vi "Single Class_Multiple_State_Self.vi"(0 "State#":i32=1000, 1 "State_Interval_Time(s)":dbl=0.001 min=0.0 max=86400.0 format="%#_13p", 2 "Time Target (s)":dbl=30.0 format="%#_13g", 3 "System_Delay(s)":dbl=0.01 min=0.0 max=86400.0 format="%#_13p") -> ()   [LabVIEW 2021]
uses:
  C:/Program Files (x86)/Hyper State Machine Framework/SSW_Hyper_State_Machine.lvlibp/State_Machine_Class/Main_State_Machine/Hyper_State_Machine.lvclass
  C:/Program Files (x86)/Hyper State Machine Framework/SSW_Hyper_State_Machine.lvlibp/State_Machine_Class/State_Machine_Module.llb/State Machine[].ctl
  C:/Program Files (x86)/Hyper State Machine Framework/SSW_Hyper_State_Machine.lvlibp/State_Machine_Class/State_Machine_Module.llb/Iterval.ctl
  C:/Program Files (x86)/Hyper State Machine Framework/SSW_Hyper_State_Machine.lvlibp/State_Machine_Class/State_Machine_Module.llb/Lock_Unlock.ctl
  C:/Program Files (x86)/Hyper State Machine Framework/SSW_Hyper_State_Machine.lvlibp
panel:
  out "Current_State_Active":bool
  out "Previous_State_Active":bool
  out "Current State":string
  out "Show_Stop_Button":bool=TRUE
  in  "Unlock":bool
  in  "Reset":bool
  in  "Lock Even":bool
  in  "Lock Odd":bool
  in  "lock All":bool
  in  "Stop":bool
  out "Timing":dbl[](array[numeric])
  out "Lock":bool[](array[boolean])
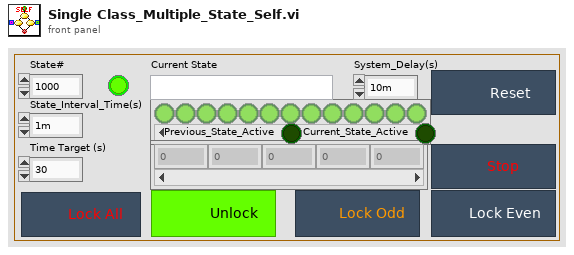
[diagram p1: front panel]
types:
  T1 = typedef "SSW_Hyper_State_Machine.lvlibp/State Machine.ctl" = cluster{"Command":string, "Data":variant}
  T2 = typedef "SSW_Hyper_State_Machine.lvlibp/State Machine[].ctl" = cluster{"Command":string, "Data":variant}[]
  T3 = typedef "SSW_Hyper_State_Machine.lvlibp/Lock_Unlock.ctl" = cluster{"Action_Mode (Get)":enum16{"Set", "Get"}, "Action_Set (False)":bool, "State_In (Wait)":string}
  T4 = typedef "SSW_Hyper_State_Machine.lvlibp/Iterval.ctl" = cluster{"Delay(s)":dbl, "State (Interval_Delay)":string}
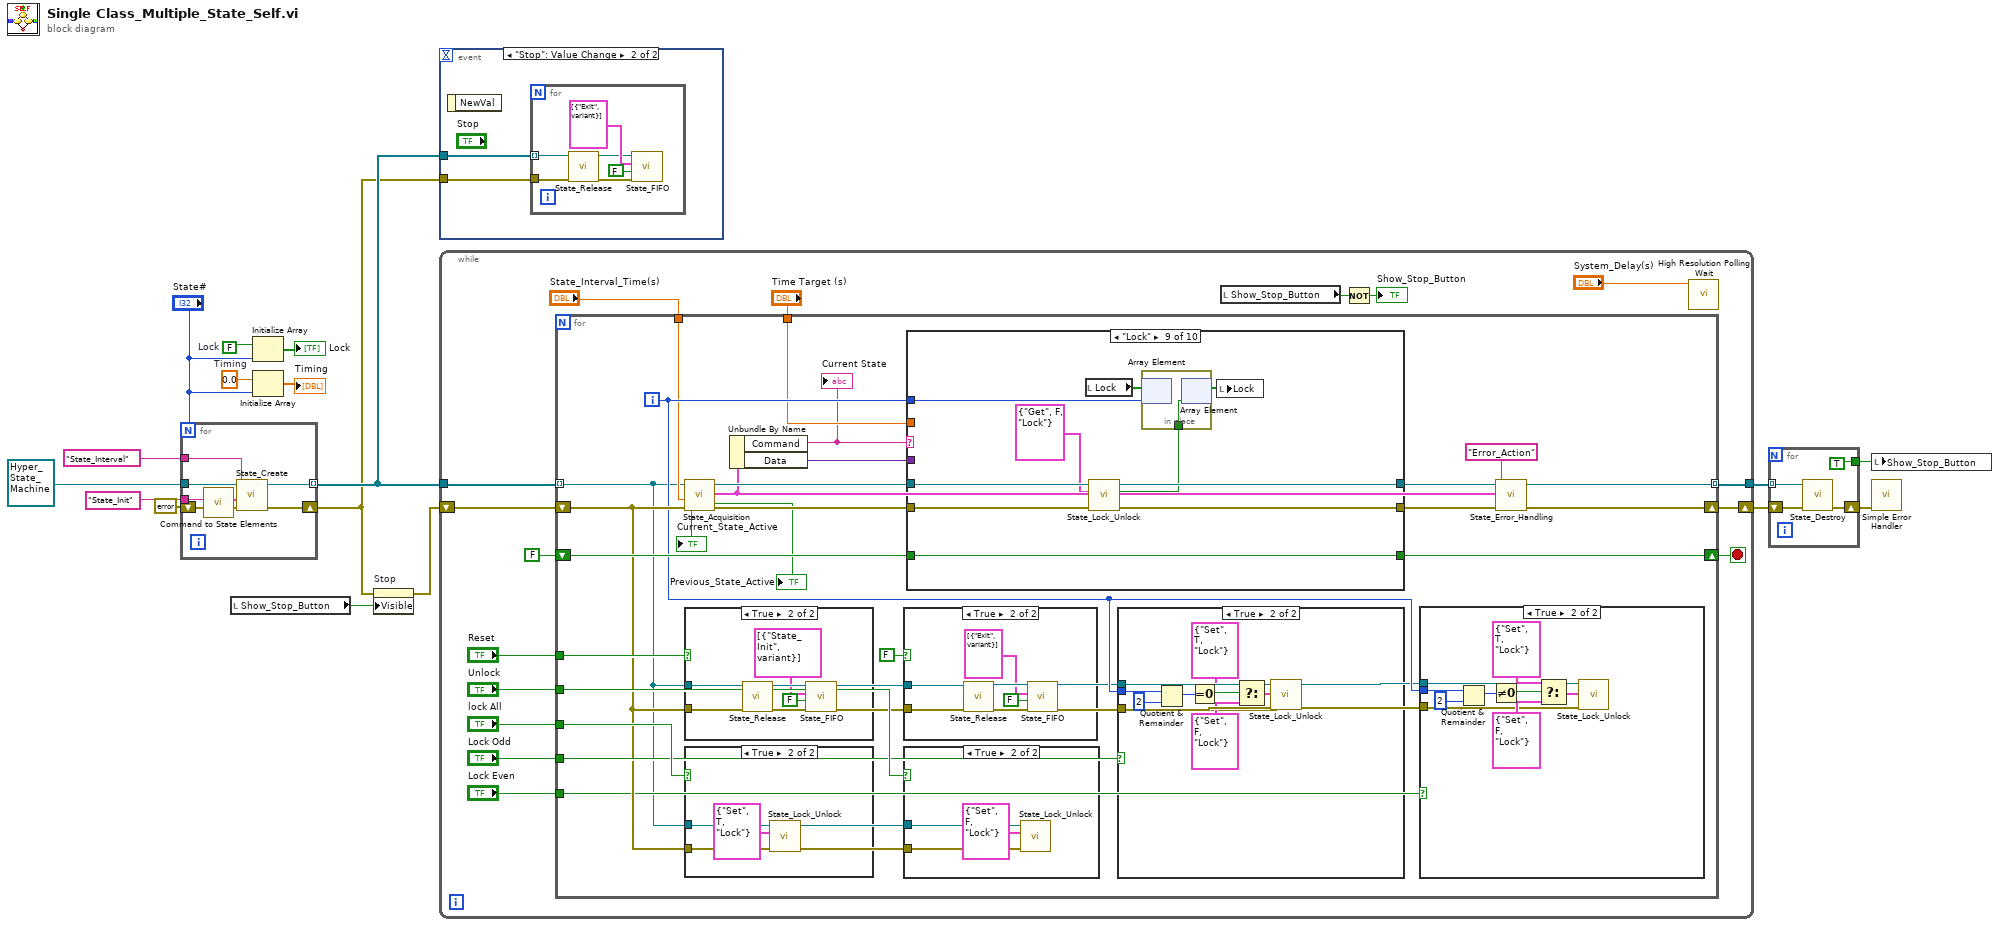
[diagram p0: block diagram]
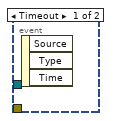
[diagram p2: hidden frame]
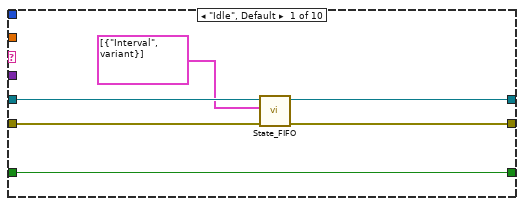
[diagram p9: hidden frame]
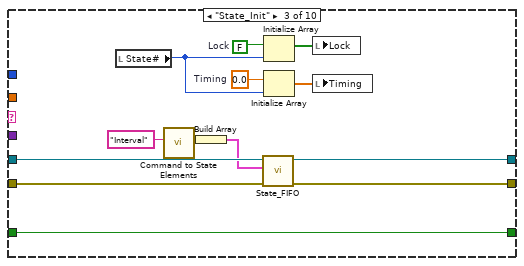
[diagram p11: hidden frame]
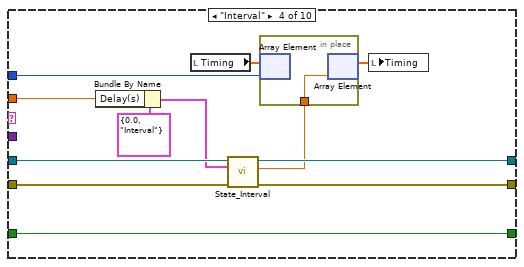
[diagram p12: hidden frame]
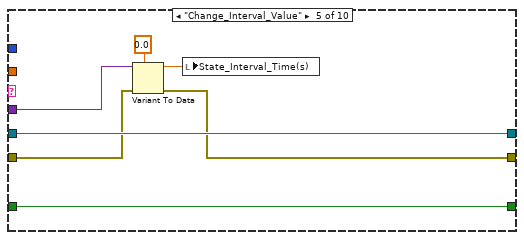
[diagram p13: hidden frame]
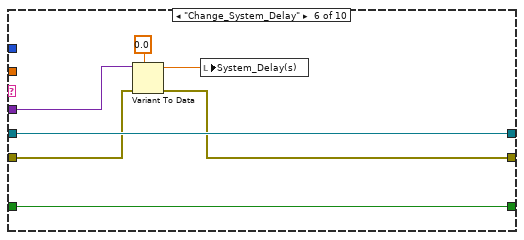
[diagram p14: hidden frame]
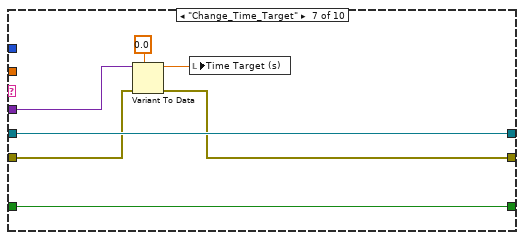
[diagram p15: hidden frame]
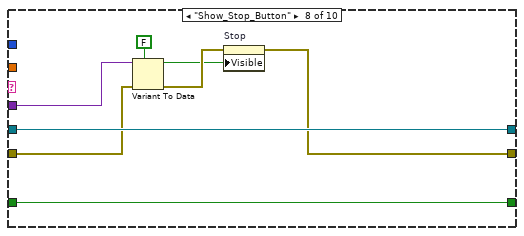
[diagram p16: hidden frame]
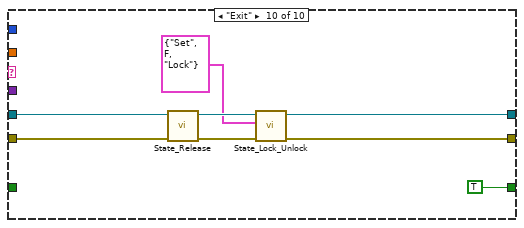
[diagram p17: hidden frame]
diagram:
  w14 = 0.0  # Timing
  w17 = FALSE  # Lock
  n1 = for {
    N: "State#" -> [_]
    tunnel: refnum<class "Hyper_State_Machine.lvclass"> refnum ("SSW_Hyper_State_Machine.lvlibp:Hyper_State_Machine.lvclass") -> [w18]
    tunnel: "State_Init" ("Command") -> [w23]
    tunnel: "State_Interval" ("Core_Interval_Name(State_Interval)") -> [w22]
    shift-right: [w21] -> w5
    shift-left: errorcluster {"status"=FALSE, "code"=0, "source"=""} ("error out") -> [w20]
    tunnel: [w19] -> w6 mode=indexing
    n2 = call "Command to State Elements.vi"("Command"=w23) -> ("Command to State Elements"=w24:T1)  [unwired: 10 in]
    n3 = call-dynamic "State_Create.vi"("error in (no error)"=w20, "Init_State(Option)"=w24, "State_Interval_Name"=w22, "State_Machine_Class in"=w18) -> ("error out"=w21:errorcluster, "State_Machine_Class out"=w19:refnum<class "Hyper_State_Machine.lvclass">)  [unwired: 5 in, 1 out]
  }
  n4 = local read "Show_Stop_Button"() -> (w8:bool)
  n5 = Initialize Array(w17, "State#") -> (→"Lock":bool[])
  n6 = Initialize Array(w14, "State#") -> (→"Timing":dbl[])
  n7 = property on="Stop" class="Bool"(error in=w5, "Visible"=w8) -> (error out=w9:errorcluster)  [unwired: 1 in, 1 out]
  n8 = event shown="[1] \"Stop\": Value Change" {
    selector: _ -> [_ _]
    dyn-events: _ -> [_ _]
    timeout: _ -> [_ _]
    tunnel: w6 -> [_ w26]
    tunnel: w5 -> [_ w25]
    event Timeout {
      n9 = event-data() -> ()  [unwired: 1 in, 3 out]
    }
    event "Stop": Value Change {
      n10 = event-data() -> ()  [unwired: 1 in, 1 out]
      n11 = for {
        tunnel: w26 -> [w28] mode=indexing
        tunnel: w25 -> [w27]
        n12 = call-dynamic "State_Release.vi"("error in (no error)"=w27, "State_Machine_Class in"=w28) -> ("error out"=w30:errorcluster, "State_Machine_Class out"=w29:refnum<class "Hyper_State_Machine.lvclass">)  [unwired: 8 in]
        n13 = call-dynamic "State_FIFO.vi"("error in (no error)"=w30, "State_Interval(Enable)"=FALSE, "State Machine[]"=T2 [{"Command"="Exit", "Data"=variant}], "State_Machine_Class in"=w29) -> ()  [unwired: 6 in, 2 out]
      }
    }
  }
  n14 = while {
    tunnel: w6 -> [w48]
    tunnel: [w44] -> w11
    shift-right: [w43] -> w10
    shift-left: w9 -> [w47]
    stop <- w46 stop-if-true
    n15 = for {
      tunnel: w48 -> [w49] mode=indexing
      shift-right: [w70] -> w43
      shift-left: w47 -> [w58]
      shift-right: [w65] -> w46
      shift-left: FALSE -> [w64]
      tunnel: [w63] -> w44 mode=indexing
      tunnel: "Reset" -> [w62]
      tunnel: "lock All" -> [w61]
      tunnel: "Unlock" -> [w60]
      tunnel: "Lock Odd" -> [w59]
      tunnel: "Lock Even" -> [w57]
      tunnel: "Time Target (s)" -> [w55]
      tunnel: "State_Interval_Time(s)" -> [w54]
      i -> [w56]
      n16 = call-dynamic "State_Acquisition.vi"("error in (no error)"=w58, "State_Interval_Time(s)"=w54, "Main_Machine_State_Class in"=w49) -> ("error out"=w71:errorcluster, "State"=w69:T1, "Main_Machine_State_Class out"=w72:refnum<class "Hyper_State_Machine.lvclass">, "Previous_State_Active"=→"Previous_State_Active":bool, "Current_State_Active"=→"Current_State_Active":bool)  [unwired: 2 in, 2 out]
      n17 = case shown="True" w62 {
        tunnel: w49 -> [_ w109]
        tunnel: w58 -> [_ w105]
        frame False {
        }
        frame True {
          n18 = call-dynamic "State_Release.vi"("error in (no error)"=w105, "State_Machine_Class in"=w109) -> ("error out"=w107:errorcluster, "State_Machine_Class out"=w108:refnum<class "Hyper_State_Machine.lvclass">)  [unwired: 8 in]
          n19 = call-dynamic "State_FIFO.vi"("error in (no error)"=w107, "State_Interval(Enable)"=FALSE, "State Machine[]"=T2 [{"Command"="State_Init", "Data"=variant}], "State_Machine_Class in"=w108) -> ()  [unwired: 6 in, 2 out]
        }
      }
      n20 = case shown="True" w61 {
        tunnel: w49 -> [_ w97]
        tunnel: w58 -> [_ w96]
        frame False {
        }
        frame True {
          n21 = call-dynamic "State_Lock_Unlock.vi"("error in (no error)"=w96, "Parameter"=T3 {"Action_Mode (Get)"=enum."Set", "Action_Set (False)"=TRUE, "State_In (Wait)"="Lock"}, "State_Machine_Class in"=w97) -> ()  [unwired: 6 in, 3 out]
        }
      }
      n22 = Unbundle By Name(w69) -> ("Command"=w52:string, "Data"=w73:variant)
      "Current State" <- w52
      n23 = case shown="True" FALSE {
        tunnel: w49 -> [_ w103]
        tunnel: w58 -> [_ w99]
        frame False {
        }
        frame True {
          n24 = call-dynamic "State_Release.vi"("error in (no error)"=w99, "State_Machine_Class in"=w103) -> ("error out"=w101:errorcluster, "State_Machine_Class out"=w102:refnum<class "Hyper_State_Machine.lvclass">)  [unwired: 8 in]
          n25 = call-dynamic "State_FIFO.vi"("error in (no error)"=w101, "State_Interval(Enable)"=FALSE, "State Machine[]"=T2 [{"Command"="Exit", "Data"=variant}], "State_Machine_Class in"=w102) -> ()  [unwired: 6 in, 2 out]
        }
      }
      n26 = case shown="True" w60 {
        tunnel: w49 -> [_ w93]
        tunnel: w58 -> [_ w94]
        frame False {
        }
        frame True {
          n27 = call-dynamic "State_Lock_Unlock.vi"("error in (no error)"=w94, "Parameter"=T3 {"Action_Mode (Get)"=enum."Set", "Action_Set (False)"=FALSE, "State_In (Wait)"="Lock"}, "State_Machine_Class in"=w93) -> ()  [unwired: 6 in, 3 out]
        }
      }
      n28 = case shown="\"Lock\"" w52 {
        tunnel: w73 -> [_ _ _ _ w150 w157 w164 w172 _ _]
        tunnel: w72 -> [w114 w118 w130 w137 w151 w158 w165 w173 w183 w191]
        tunnel: w71 -> [w113 w117 w128 w136 w149 w156 w163 w171 w182 w190]
        tunnel: [w112 w118 w129 w134 w151 w158 w165 w173 w181 w187] -> w67
        tunnel: [w111 w117 w127 w133 w148 w155 w162 w166 w180 w186] -> w66
        tunnel: w56 -> [_ _ _ w143 _ _ _ _ w176 _]
        tunnel: [w115 w116 w131 w140 w146 w153 w160 w170 w178 TRUE] -> w65
        tunnel: w64 -> [w115 w116 w131 w140 w146 w153 w160 w170 w178 _]
        tunnel: w55 -> [_ _ _ w139 _ _ _ _ _ _]
        frame "Idle", Default {
          n29 = call-dynamic "State_FIFO.vi"("error in (no error)"=w113, "State Machine[]"=T2 [{"Command"="Interval", "Data"=variant}], "State_Machine_Class in"=w114) -> ("error out"=w111:errorcluster, "State_Machine_Class out"=w112:refnum<class "Hyper_State_Machine.lvclass">)  [unwired: 7 in]
        }
        frame "State_Interval" {
          # "Execute Every Define of State Interval Time"
        }
        frame "State_Init" {
          w123 = 0.0  # Timing
          w122 = FALSE  # Lock
          n30 = local read "State#"() -> (w121:i32)
          n31 = call "Command to State Elements.vi"("Command"="Interval") -> ("Command to State Elements"=w125:T1)  [unwired: 10 in]
          n32 = Build Array(w125) -> (w124:T1[])
          n33 = call-dynamic "State_FIFO.vi"("error in (no error)"=w128, "State Machine[]"=w124, "State_Machine_Class in"=w130) -> ("error out"=w127:errorcluster, "State_Machine_Class out"=w129:refnum<class "Hyper_State_Machine.lvclass">)  [unwired: 7 in]
          n34 = Initialize Array(w122, w121) -> (w119:bool[])
          n35 = Initialize Array(w123, w121) -> (w120:dbl[])
          n36 = local write "Lock"(w119) -> ()
          n37 = local write "Timing"(w120) -> ()
        }
        frame "Interval" {
          n38 = Bundle By Name(cluster=T4 {"Delay(s)"=0.0, "State (Interval_Delay)"="Interval"} ("Parameter"), "Delay(s)"=w139) -> (w135:T4)
          n39 = local read "Timing"() -> (w142:dbl[])
          n40 = call-dynamic "State_Interval.vi"("error in (no error)"=w136, "Parameter"=w135, "State_Machine_Class in"=w137) -> ("error out"=w133:errorcluster, "Elapsed Time(s)"=w132:dbl, "State_Machine_Class out"=w134:refnum<class "Hyper_State_Machine.lvclass">)  [unwired: 6 in]
          n41 = in-place {
            in-place-border: w132 -> [w144]
            n42 = in-place-array #1(w142, w143) -> ()  [unwired: 1 out]
            n43 = in-place-array #1(w144) -> (w141:dbl[])  [unwired: 1 out]
          }
          n44 = local write "Timing"(w141) -> ()
        }
        frame "Change_Interval_Value" {
          n45 = Variant To Data(error in=w149, type=0.0 ("Time Target (s)"), Variant=w150) -> (data=w145:dbl, error out=w148:errorcluster)
          n46 = local write "State_Interval_Time(s)"(w145) -> ()
        }
        frame "Change_System_Delay" {
          n47 = Variant To Data(error in=w156, type=0.0 ("Time Target (s)"), Variant=w157) -> (data=w152:dbl, error out=w155:errorcluster)
          n48 = local write "System_Delay(s)"(w152) -> ()
        }
        frame "Change_Time_Target" {
          n49 = Variant To Data(error in=w163, type=0.0 ("Time Target (s)"), Variant=w164) -> (data=w159:dbl, error out=w162:errorcluster)
          n50 = local write "Time Target (s)"(w159) -> ()
        }
        frame "Show_Stop_Button" {
          n51 = Variant To Data(error in=w171, type=FALSE, Variant=w172) -> (data=w167:bool, error out=w168:errorcluster)
          n52 = property on="Stop" class="Bool"(error in=w168, "Visible"=w167) -> (error out=w166:errorcluster)  [unwired: 1 in, 1 out]
        }
        frame "Lock" {
          n53 = local read "Lock"() -> (w174:bool[])
          n54 = call-dynamic "State_Lock_Unlock.vi"("error in (no error)"=w182, "Parameter"=T3 {"Action_Mode (Get)"=enum."Get", "Action_Set (False)"=FALSE, "State_In (Wait)"="Lock"}, "State_Machine_Class in"=w183) -> ("error out"=w180:errorcluster, "Action_Get"=w175:bool, "State_Machine_Class out"=w181:refnum<class "Hyper_State_Machine.lvclass">)  [unwired: 6 in]
          n55 = in-place {
            in-place-border: w175 -> [w184]
            n56 = in-place-array #2(w174, w176) -> ()  [unwired: 1 out]
            n57 = in-place-array #2(w184) -> (w177:bool[])  [unwired: 1 out]
          }
          n58 = local write "Lock"(w177) -> ()
        }
        frame "Exit" {
          n59 = call-dynamic "State_Release.vi"("error in (no error)"=w190, "State_Machine_Class in"=w191) -> ("error out"=w188:errorcluster, "State_Machine_Class out"=w189:refnum<class "Hyper_State_Machine.lvclass">)  [unwired: 8 in]
          n60 = call-dynamic "State_Lock_Unlock.vi"("error in (no error)"=w188, "Parameter"=T3 {"Action_Mode (Get)"=enum."Set", "Action_Set (False)"=FALSE, "State_In (Wait)"="Lock"}, "State_Machine_Class in"=w189) -> ("error out"=w186:errorcluster, "State_Machine_Class out"=w187:refnum<class "Hyper_State_Machine.lvclass">)  [unwired: 6 in, 1 out]
        }
      }
      n61 = case shown="True" w59 {
        tunnel: w56 -> [_ w85]
        tunnel: w49 -> [_ w84]
        tunnel: w58 -> [_ w83]
        frame False {
        }
        frame True {
          n62 = Quotient & Remainder(x=w85, y=2) -> (x-y*floor(x/y)=w90:i32)  [unwired: 1 out]
          n63 = Equal To 0?(x=w90) -> (x = 0?=w89:bool)
          n64 = Select(t=T3 {"Action_Mode (Get)"=enum."Set", "Action_Set (False)"=TRUE, "State_In (Wait)"="Lock"} ("Parameter"), s=w89, f=T3 {"Action_Mode (Get)"=enum."Set", "Action_Set (False)"=FALSE, "State_In (Wait)"="Lock"} ("Parameter")) -> (s? t:f=w86:T3)
          n65 = call-dynamic "State_Lock_Unlock.vi"("error in (no error)"=w83, "Parameter"=w86, "State_Machine_Class in"=w84) -> ()  [unwired: 6 in, 3 out]
        }
      }
      n66 = case shown="True" w57 {
        tunnel: w56 -> [_ w76]
        tunnel: w49 -> [_ w75]
        tunnel: w58 -> [_ w74]
        frame False {
        }
        frame True {
          n67 = Quotient & Remainder(x=w76, y=2) -> (x-y*floor(x/y)=w81:i32)  [unwired: 1 out]
          n68 = Not Equal To 0?(x=w81) -> (x != 0?=w80:bool)
          n69 = Select(t=T3 {"Action_Mode (Get)"=enum."Set", "Action_Set (False)"=TRUE, "State_In (Wait)"="Lock"} ("Parameter"), s=w80, f=T3 {"Action_Mode (Get)"=enum."Set", "Action_Set (False)"=FALSE, "State_In (Wait)"="Lock"} ("Parameter")) -> (s? t:f=w77:T3)
          n70 = call-dynamic "State_Lock_Unlock.vi"("error in (no error)"=w74, "Parameter"=w77, "State_Machine_Class in"=w75) -> ()  [unwired: 6 in, 3 out]
        }
      }
      n71 = call-dynamic "State_Error_Handling.vi"("error in (no error)"=w66, "Reply_State_Name"="Error_Action", "Handling_State(State_Acquisition)"=w69, "State_Machine_Class in"=w67) -> ("error out"=w70:errorcluster, "State_Machine_Class out"=w63:refnum<class "Hyper_State_Machine.lvclass">)  [unwired: 6 in]
    }
    n72 = local read "Show_Stop_Button"() -> (w34:bool)
    n73 = Not(x=w34) -> (.not. x?=→"Show_Stop_Button":bool)
    n74 = call <vilib>:"High Resolution Polling Wait.vi"("seconds to wait"="System_Delay(s)") -> ()  [unwired: 10 in, 1 out]
  }
  n75 = for {
    shift-right: [w196] -> w12
    shift-left: w10 -> [w195]
    tunnel: w11 -> [w194] mode=indexing
    tunnel: [TRUE ("Show_Stop_Button")] -> w7
    n76 = call-dynamic "State_Destroy.vi"("error in (no error)"=w195, "State_Machine_Class in"=w194) -> ("error out"=w196:errorcluster)  [unwired: 9 in]
  }
  n77 = local write "Show_Stop_Button"(w7) -> ()
  n78 = call <vilib>:"Simple Error Handler.vi"("error in (no error)"=w12) -> ()  [unwired: 4 in, 5 out]
